vi "Stacking SSS.vi"(7 "Robot Controls":T1, 11 "Actuator Values in":T2) -> (3 "Actuator Values Out":T2)   [LabVIEW 2014]
uses:
  Stacking SS Actuators.ctl
  <vilib>/Rock Robotics/WPI/Solenoid/WPI_SolenoidValue.ctl
  Robot Commands.ctl
  Global Variables/Settings.vi
  Global Variables/Sensor Data (Edited).vi
panel:
  in  "Time when Arm Last Moved":dbl format="%#_13g"
  # "Field Centric"
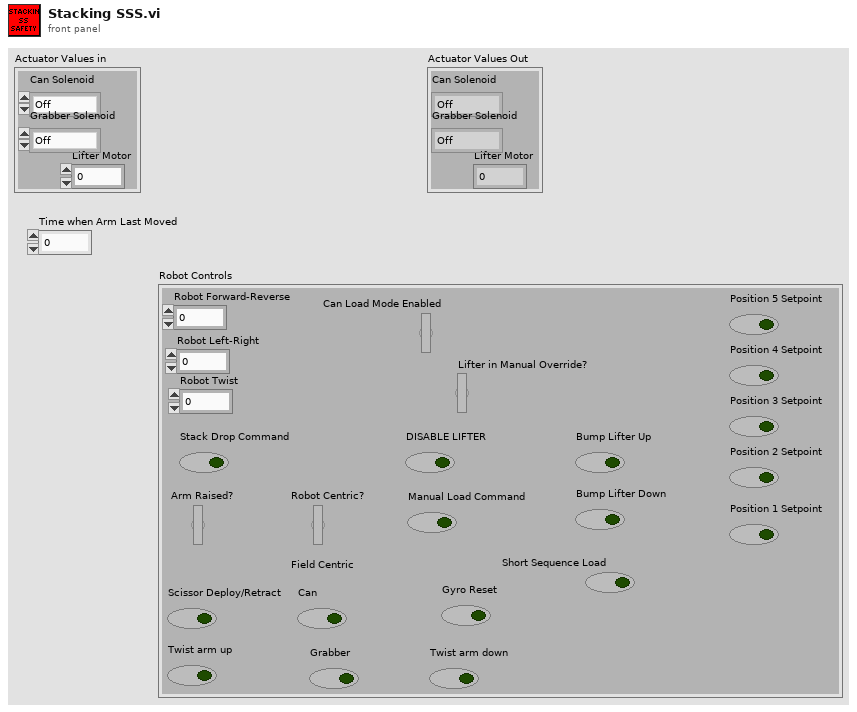
[diagram p1: front panel]
types:
  T1 = typedef "Robot Commands.ctl" = cluster{"Robot Forward-Reverse":dbl, "Robot Left-Right":dbl, "Robot Twist":dbl, "Can Load Mode Enabled":bool, "Lifter in Manual Override?":bool, "Stack Drop Command":bool, "Arm Raised?":bool, "DISABLE LIFTER":bool, "Position 1 Setpoint":bool, "Position 2 Setpoint":bool, "Position 3 Setpoint":bool, "Position 4 Setpoint":bool, "Position 5 Setpoint":bool, "Bump Lifter Down":bool, "Bump Lifter Up":bool, "Manual Load Command":bool, "Robot Centric?":bool, "Scissor Deploy/Retract":bool, "Grabber":bool, "Can":bool, "Twist arm up":bool, "Gyro Reset":bool, "Twist arm down":bool, "Short Sequence Load":bool}
  T2 = typedef "Stacking SS Actuators.ctl" = cluster{"Can Solenoid":T3, "Lifter Motor":dbl, "Grabber Solenoid":T3}
  T3 = typedef "WPI_SolenoidValue.ctl" = enum16{"Off", "On", "Forward", "Reverse"}
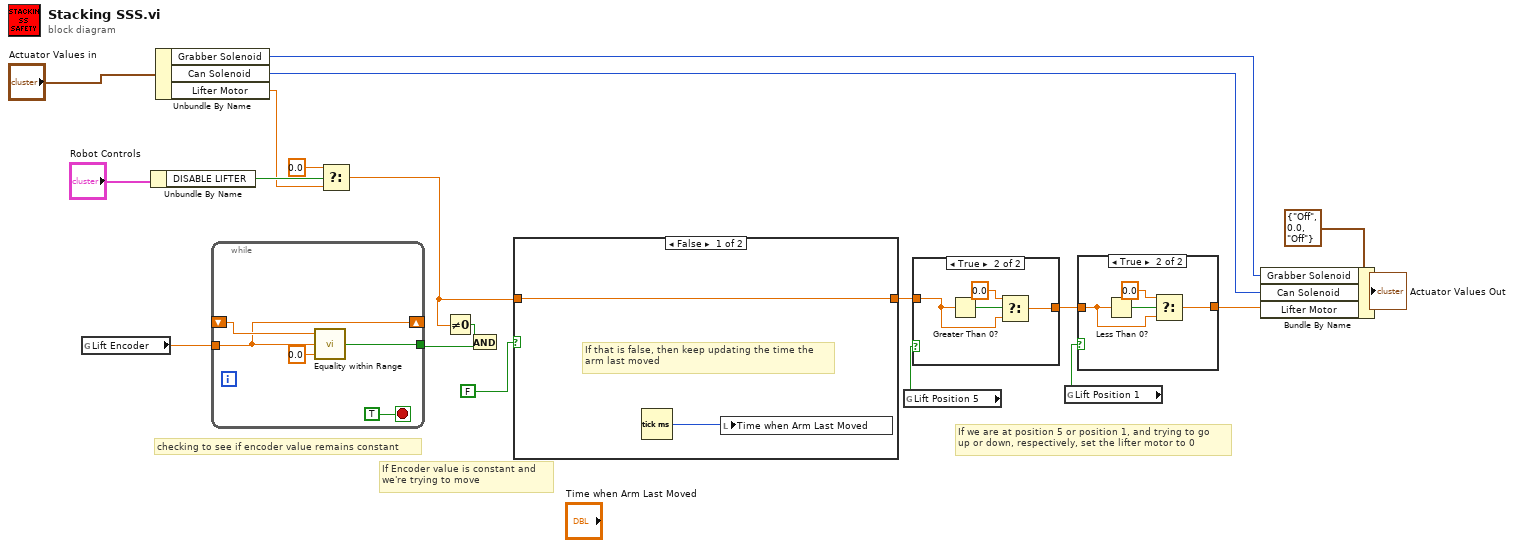
[diagram p0: block diagram]
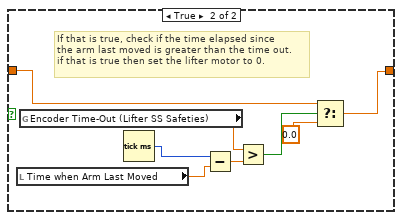
[diagram p2: hidden frame]
diagram:
  # "If we are at position 5 or position 1, and trying to go\nup or down, respectively, set the lifter motor to 0"
  # "If Encoder value is constant and \nwe're trying to move"
  # "checking to see if encoder value remains constant"
  n1 = global read "Sensor Data (Edited).vi" "Lift Encoder"() -> (w10:dbl)
  n2 = Unbundle By Name("Robot Controls") -> ("DISABLE LIFTER"=w4:bool)
  n3 = Unbundle By Name("Actuator Values in") -> ("Grabber Solenoid"=w6:T3, "Can Solenoid"=w11:T3, "Lifter Motor"=w2:dbl)
  n4 = while {
    tunnel: [w20] -> w13
    shift-right: [w22] -> _
    shift-left: _ -> [w23]
    tunnel: w10 -> [w22]
    stop <- TRUE stop-if-true
    n5 = call "Equality within Range.vi"("Range"=0.0, "Y"=w22, "X"=w23) -> ("X = Y within Range?"=w20:bool)
  }
  n6 = Select(t=0.0, s=w4, f=w2) -> (s? t:f=w3:dbl)
  n7 = Not Equal To 0?(x=w3) -> (x != 0?=w14:bool)
  n8 = And(x=w14, y=w13) -> ()  [unwired: 1 out]
  n9 = case shown="False" FALSE {
    tunnel: w3 -> [w26 w31]
    tunnel: [w26 w30] -> w17
    frame False {
      # "If that is false, then keep updating the time the \narm last moved"
      n10 = Tick Count (ms)() -> (millisecond timer value=w25:u32)
      n11 = local write "Time when Arm Last Moved"(w25) -> ()
    }
    frame True {
      # "If that is true, check if the time elapsed since\nthe arm last moved is greater than the time out.\nif that is true then set the lifter motor to 0."
      n12 = local read "Time when Arm Last Moved"() -> (w29:dbl)
      n13 = global read "Settings.vi" "Encoder Time-Out (Lifter SS Safeties)"() -> (w27:dbl)
      n14 = Tick Count (ms)() -> (millisecond timer value=w28:u32)
      n15 = Subtract(x=w28, y=w29) -> (x-y=w34:dbl)
      n16 = Greater?(x=w27, y=w34) -> (0:w32:bool)
      n17 = Select(t=w31, s=w32, f=0.0) -> (s? t:f=w30:dbl)
    }
  }
  n18 = global read "Sensor Data (Edited).vi" "Lift Position 5"() -> (w9:bool)
  n19 = case shown="True" w9 {
    tunnel: [w35 w38] -> w19
    tunnel: w17 -> [w35 w36]
    frame False {
    }
    frame True {
      n20 = Greater Than 0?(x=w36) -> (x > 0?=w39:bool)
      n21 = Select(t=0.0 ("f"), s=w39, f=w36) -> (s? t:f=w38:dbl)
    }
  }
  n22 = global read "Sensor Data (Edited).vi" "Lift Position 1"() -> (w8:bool)
  n23 = case shown="True" w8 {
    tunnel: w19 -> [w40 w41]
    tunnel: [w40 w43] -> w12
    frame False {
    }
    frame True {
      n24 = Less Than 0?(x=w41) -> (x < 0?=w44:bool)
      n25 = Select(t=0.0 ("f"), s=w44, f=w41) -> (s? t:f=w43:dbl)
    }
  }
  n26 = Bundle By Name(cluster=T2 {"Can Solenoid"=enum."Off", "Lifter Motor"=0.0, "Grabber Solenoid"=enum."Off"} ("Actuator Values Out"), "Grabber Solenoid"=w6, "Can Solenoid"=w11, "Lifter Motor"=w12) -> (→"Actuator Values Out":T2)
